vi "Update FIU.vi"(8 "error in":errorcluster, 10 "FIU SPI command":T1, 11 "DMA FIFO ref":refnum<k20>) -> (0 "error out":errorcluster, 2 "FIU SPI command out":T1)   [LabVIEW 2014]
uses:
  Shared/Type Defs/FIU compiled.ctl
  <vilib>/NI Veristand/Custom Device API/Global Data Refs.vi
  <vilib>/Utility/error.llb/Error Cluster From Error Code.vi
  <vilib>/rvi/errors/niLvFpgaAdjustHostInterfaceError.vi
  <vilib>/rvi/interface/nirviMethod/nirviMethod.xnode
  <vilib>/NI Veristand/Custom Device API/Custom Device API.lvlib
  Shared/SLSC configuration Shared.lvlib
  <vilib>/FPGAPlugInAG/Dynamic/niLvFpga_WriteFifo_Dynamic.vi
  <vilib>/rvi/errors/niLvFpgaMergeErrorWithErrorCode.vi
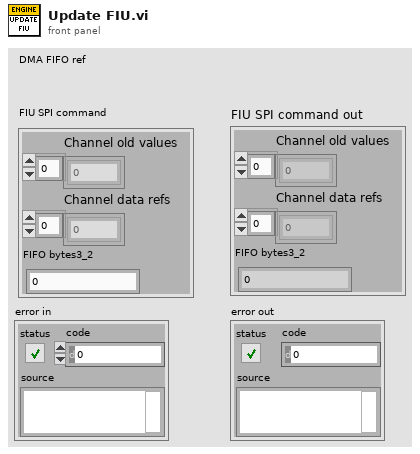
[diagram p1: front panel]
types:
  T1 = typedef "SLSC configuration Shared.lvlib/FIU compiled.ctl" = cluster{"Channel old values":dbl[], "Channel data refs":i32[], "FIFO bytes3_2":u16}
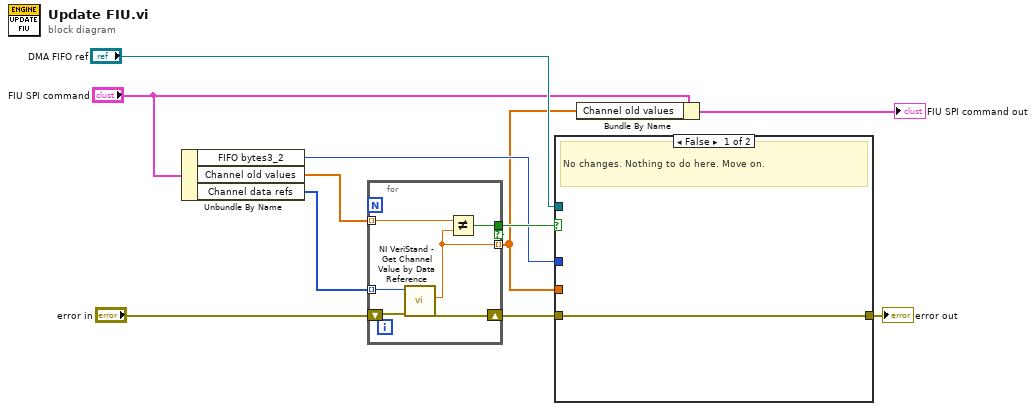
[diagram p0: block diagram]
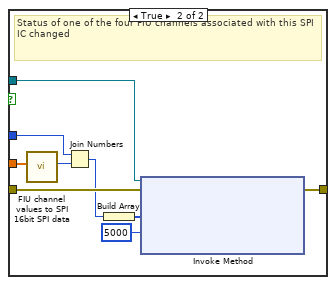
[diagram p2: hidden frame]
diagram:
  n1 = Unbundle By Name("FIU SPI command") -> ("FIFO bytes3_2"=w7:u16, "Channel old values"=w9:dbl[], "Channel data refs"=w11:i32[])
  n2 = for {
    tunnel: w11 -> [w17] mode=indexing
    shift-right: [w15] -> w5
    shift-left: "error in" -> [w16]
    tunnel: w9 -> [w14] mode=indexing
    tunnel: [w13] -> w3 mode=indexing
    tunnel: [w12] -> w8 if=w12
    n3 = call <vilib>:"NI VeriStand - Get Channel Value by Data Reference.vi"("error in (no error)"=w16, "Data Reference in"=w17) -> ("error out"=w15:errorcluster, "Value"=w13:dbl)  [unwired: 8 out]
    n4 = Not Equal?(x=w14, y=w13) -> (x != y?=w12:bool)
  }
  n5 = case shown="False" w8 {
    tunnel: w3 -> [_ w27]
    tunnel: w7 -> [_ w26]
    tunnel: "DMA FIFO ref" -> [_ w23]
    tunnel: w5 -> [w18 w24]
    tunnel: [w18 w19] -> w1
    frame False {
      # "No changes. Nothing to do here. Move on."
    }
    frame True {
      # "Status of one of the four FIU channels associated with this SPI IC changed"
      n6 = call "FIU channel values to SPI 16bit SPI data.vi"("FIU Channel values"=w27) -> ("data word"=w25:u16)  [unwired: 10 in]
      n7 = Join Numbers(hi=w26, lo=w25) -> ((hi.lo)=w22:u32)
      n8 = Build Array(w22) -> (w21:u32[])
      n9 = xnode "Invoke Method"("FPGA VI Reference In"=w23, "error in"=w24, "Data"=w21, "Timeout (ms)"=5000) -> ("error out"=w19:errorcluster)  [unwired: 2 out]
    }
  }
  "error out" <- w1
  n10 = Bundle By Name(cluster="FIU SPI command", "Channel old values"=w3) -> (→"FIU SPI command out":T1)
